vi "AnalogInput_mic.vi"   [LabVIEW 2014]
uses:
  <vilib>/eio/EIONode/EIONode.xnode
  <vilib>/rvi/eio/common/nirviEmuTemplateMethod_errors.vi
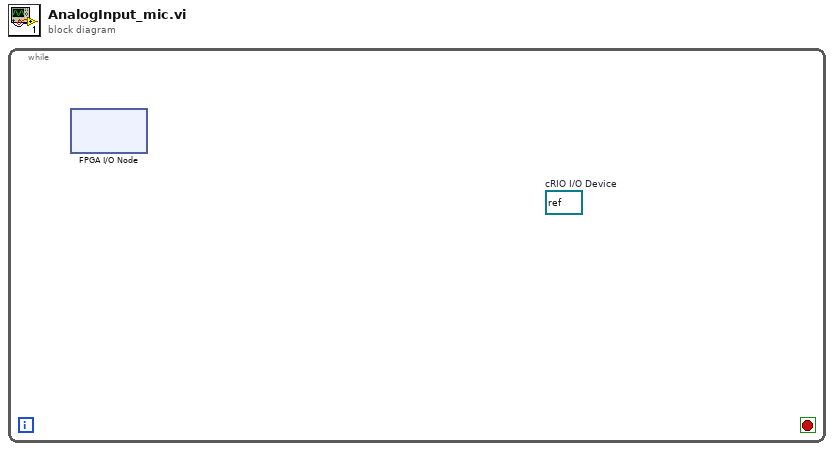
[diagram p0: block diagram]
diagram:
  n1 = while {
    stop <- _ stop-if-true
    (unwired) refnum<k21> refnum  # cRIO I/O Device
    n2 = xnode "FPGA I/O Node"() -> ()  [unwired: 1 in, 2 out]
  }
